vi "Close Local Event Log.vi"(8 "error in (no error)":errorcluster, 10 "Deferred Close Time (0 ms)":u32, 11 "Log Instance":refnum<class "LoggerReference.lvclass">) -> (0 "error out":errorcluster)   [LabVIEW 2020, in "MVA Framework.lvlib" / "Composed Log.lvlib" / "LoggerReference.lvclass"]
doc: "Close the local event log. If a deferred close time is defined, an asynchronous timer will be used to defer closing the log. Use this feature in a multi threaded applications where some modules may not be fully stopped when the close call occurs."
uses:
  LoggerReference.lvclass
  LoggerReference.lvclass/LoggerReference.ctl
  Deferred Stop.vi
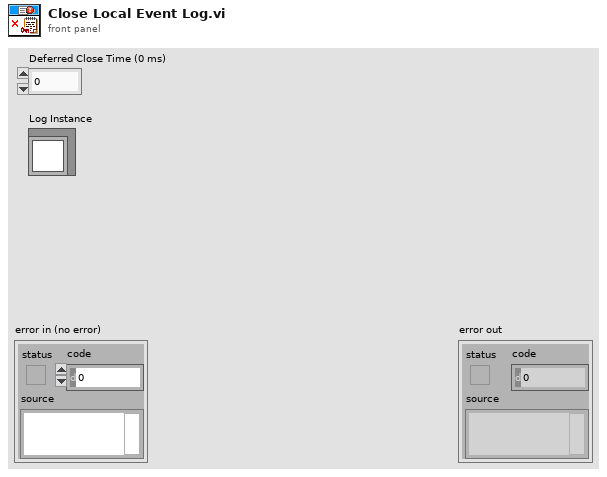
[diagram p1: front panel]
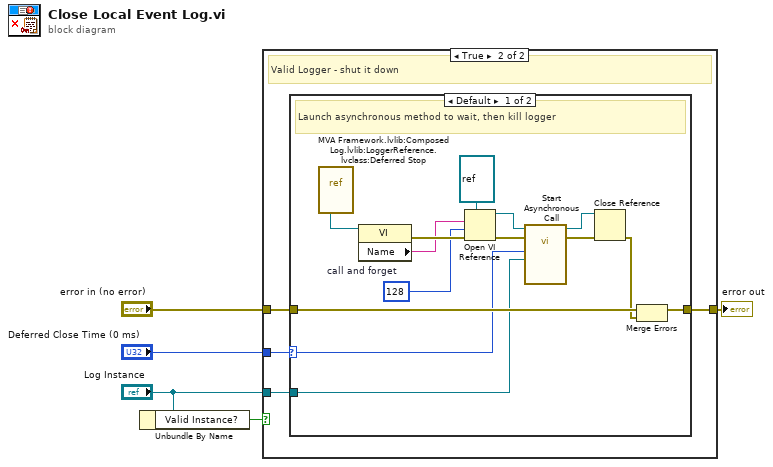
[diagram p0: block diagram]
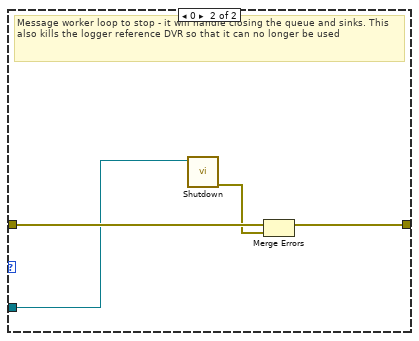
[diagram p3: hidden frame]
diagram:
  n1 = Unbundle By Name("Log Instance") -> ("Valid Instance?"=w1:bool)
  n2 = case shown="True" w1 {
    tunnel: [w6 w10] -> w5
    tunnel: "error in (no error)" -> [w6 w9]
    tunnel: "Deferred Close Time (0 ms)" -> [_ w8]
    tunnel: "Log Instance" -> [_ w7]
    frame False {
      # "Not a valid log - do nothing"
    }
    frame True {
      # "Valid Logger - shut it down"
      n3 = case shown="Default" w8 {
        selector: w8 -> [w12 _]
        tunnel: w9 -> [w24 w28]
        tunnel: [w14 w27] -> w10
        tunnel: w7 -> [w11 w26]
        frame Default {
          w15 = 128  # call and forget
          # "Launch asynchronous method to wait, then kill logger"
          n4 = vi-ref "MVA Framework.lvlib:Composed Log.lvlib:LoggerReference.lvclass:Deferred Stop.vi"() -> (w23:refnum<vi>)
          n5 = property class="VI"(reference=w23) -> (error out=w22:errorcluster, "Name"=w20:string)  [unwired: 1 in, 1 out]
          n6 = Open VI Reference(type specifier VI Refnum (for type only)=refnum<vi> refnum, vi path=w20, options=w15, error in (no error)=w22) -> (vi reference=w18:refnum<vi>, error out=w19:errorcluster)  [unwired: 2 in]
          n7 = call-by-ref "Start Asynchronous Call"(reference=w18, error in=w19, "Log Instance"=w11, "Deferred Stop Time"=w12) -> (reference out=w16:refnum<vi>, error out=w17:errorcluster)  [unwired: 10 in]
          n8 = Close Reference(reference=w16, error in (no error)=w17) -> (error out=w13:errorcluster)
          n9 = Merge Errors(w24, w13) -> (w14:errorcluster)
        }
        frame 0 {
          # "Message worker loop to stop - it will handle closing the queue and sinks. This also kills the logger reference DVR so that it can no longer be used"
          n10 = call "Shutdown.vi"("LoggerReference in"=w26) -> ("error out"=w25:errorcluster)  [unwired: 10 in]
          n11 = Merge Errors(w28, w25) -> (w27:errorcluster)
        }
      }
    }
  }
  "error out" <- w5
